vi "tsfifo_receive_canfd_msgs.vi"(7 "error in (no error)":errorcluster caption="错误输入（无错误）", 8 "Display message type":u16(ring) items=["Rx", "Rx&Tx"], 9 "AAPPChannel":u32, 10 "Path":path) -> (0 "error out":errorcluster caption="错误输出", 1 "tsfifo_receive_can_msgs":i32, 2 "ACANMsgBuffer":T1(array[cluster]), 3 "Path output":path)   [LabVIEW 2014]
doc: "Function Introduction :\nReceive FIFO CAN messages\nCall location :\ninput parameter :\nACANFDBuffers: CANFD buffers\nACANFDBuffers: canfd buffer size\nAChn: Channel Index\nARxTx: READ_TX_RX_deF_ARxTx enumeration, if the value is 0, only RX messages are received; if the value is\n1. Receive TX Rx message\nReturn value :\n0: Execution successful\nOther values: Failed"
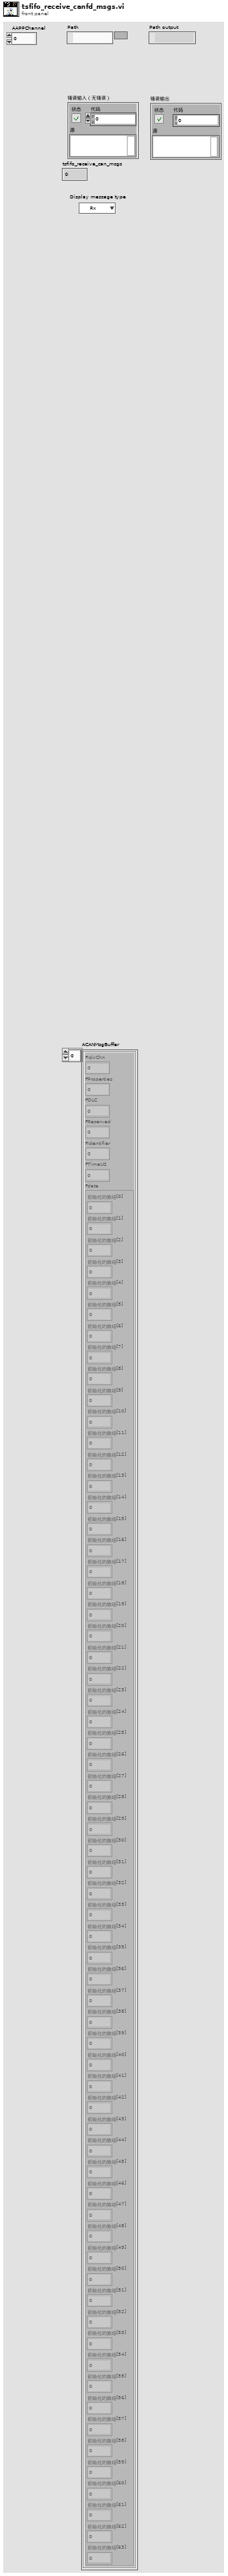
[diagram p1: front panel]
types:
  T1 = cluster{"FIdxChn":u8, "FProperties":u8, "FDLC":u8, "FReserved":u8, "FIdentifier":i32, "FTimeUS":u64, "Fdata":cluster{"初始化的数组[0]":u8, "初始化的数组[1]":u8, "初始化的数组[2]":u8, "初始化的数组[3]":u8, "初始化的数组[4]":u8, "初始化的数组[5]":u8, "初始化的数组[6]":u8, "初始化的数组[7]":u8, "初始化的数组[8]":u8, "初始化的数组[9]":u8, "初始化的数组[10]":u8, "初始化的数组[11]":u8, "初始化的数组[12]":u8, "初始化的数组[13]":u8, "初始化的数组[14]":u8, "初始化的数组[15]":u8, "初始化的数组[16]":u8, "初始化的数组[17]":u8, "初始化的数组[18]":u8, "初始化的数组[19]":u8, "初始化的数组[20]":u8, "初始化的数组[21]":u8, "初始化的数组[22]":u8, "初始化的数组[23]":u8, "初始化的数组[24]":u8, "初始化的数组[25]":u8, "初始化的数组[26]":u8, "初始化的数组[27]":u8, "初始化的数组[28]":u8, "初始化的数组[29]":u8, "初始化的数组[30]":u8, "初始化的数组[31]":u8, "初始化的数组[32]":u8, "初始化的数组[33]":u8, "初始化的数组[34]":u8, "初始化的数组[35]":u8, "初始化的数组[36]":u8, "初始化的数组[37]":u8, "初始化的数组[38]":u8, "初始化的数组[39]":u8, "初始化的数组[40]":u8, "初始化的数组[41]":u8, "初始化的数组[42]":u8, "初始化的数组[43]":u8, "初始化的数组[44]":u8, "初始化的数组[45]":u8, "初始化的数组[46]":u8, "初始化的数组[47]":u8, "初始化的数组[48]":u8, "初始化的数组[49]":u8, "初始化的数组[50]":u8, "初始化的数组[51]":u8, "初始化的数组[52]":u8, "初始化的数组[53]":u8, "初始化的数组[54]":u8, "初始化的数组[55]":u8, "初始化的数组[56]":u8, "初始化的数组[57]":u8, "初始化的数组[58]":u8, "初始化的数组[59]":u8, "初始化的数组[60]":u8, "初始化的数组[61]":u8, "初始化的数组[62]":u8, "初始化的数组[63]":u8}}[]
  T2 = cluster{"FIdxChn":u8, "FProperties":u8, "FDLC":u8, "FReserved":u8, "FIdentifier":i32, "FTimeUS":u64, "Fdata":cluster{"初始化的数组[0]":u8, "初始化的数组[1]":u8, "初始化的数组[2]":u8, "初始化的数组[3]":u8, "初始化的数组[4]":u8, "初始化的数组[5]":u8, "初始化的数组[6]":u8, "初始化的数组[7]":u8, "初始化的数组[8]":u8, "初始化的数组[9]":u8, "初始化的数组[10]":u8, "初始化的数组[11]":u8, "初始化的数组[12]":u8, "初始化的数组[13]":u8, "初始化的数组[14]":u8, "初始化的数组[15]":u8, "初始化的数组[16]":u8, "初始化的数组[17]":u8, "初始化的数组[18]":u8, "初始化的数组[19]":u8, "初始化的数组[20]":u8, "初始化的数组[21]":u8, "初始化的数组[22]":u8, "初始化的数组[23]":u8, "初始化的数组[24]":u8, "初始化的数组[25]":u8, "初始化的数组[26]":u8, "初始化的数组[27]":u8, "初始化的数组[28]":u8, "初始化的数组[29]":u8, "初始化的数组[30]":u8, "初始化的数组[31]":u8, "初始化的数组[32]":u8, "初始化的数组[33]":u8, "初始化的数组[34]":u8, "初始化的数组[35]":u8, "初始化的数组[36]":u8, "初始化的数组[37]":u8, "初始化的数组[38]":u8, "初始化的数组[39]":u8, "初始化的数组[40]":u8, "初始化的数组[41]":u8, "初始化的数组[42]":u8, "初始化的数组[43]":u8, "初始化的数组[44]":u8, "初始化的数组[45]":u8, "初始化的数组[46]":u8, "初始化的数组[47]":u8, "初始化的数组[48]":u8, "初始化的数组[49]":u8, "初始化的数组[50]":u8, "初始化的数组[51]":u8, "初始化的数组[52]":u8, "初始化的数组[53]":u8, "初始化的数组[54]":u8, "初始化的数组[55]":u8, "初始化的数组[56]":u8, "初始化的数组[57]":u8, "初始化的数组[58]":u8, "初始化的数组[59]":u8, "初始化的数组[60]":u8, "初始化的数组[61]":u8, "初始化的数组[62]":u8, "初始化的数组[63]":u8}}
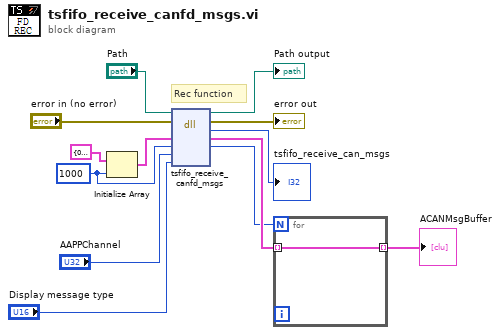
[diagram p0: block diagram]
diagram:
  w1 = 1000 ("维数大小")
  # "Rec function"
  n1 = Initialize Array(T2 {"FIdxChn"=0, "FProperties"=0, "FDLC"=0, "FReserved"=0, "FIdentifier"=0, "FTimeUS"=0, "Fdata"={"初始化的数组[0]"=0, "初始化的数组[1]"=0, "初始化的数组[2]"=0, "初始化的数组[3]"=0, "初始化的数组[4]"=0, "初始化的数组[5]"=0, "初始化的数组[6]"=0, "初始化的数组[7]"=0, "初始化的数组[8]"=0, "初始化的数组[9]"=0, "初始化的数组[10]"=0, "初始化的数组[11]"=0, "初始化的数组[12]"=0, "初始化的数组[13]"=0, "初始化的数组[14]"=0, "初始化的数组[15]"=0, "初始化的数组[16]"=0, "初始化的数组[17]"=0, "初始化的数组[18]"=0, "初始化的数组[19]"=0, "初始化的数组[20]"=0, "初始化的数组[21]"=0, "初始化的数组[22]"=0, "初始化的数组[23]"=0, "初始化的数组[24]"=0, "初始化的数组[25]"=0, "初始化的数组[26]"=0, "初始化的数组[27]"=0, "初始化的数组[28]"=0, "初始化的数组[29]"=0, "初始化的数组[30]"=0, "初始化的数组[31]"=0, "初始化的数组[32]"=0, "初始化的数组[33]"=0, "初始化的数组[34]"=0, "初始化的数组[35]"=0, "初始化的数组[36]"=0, "初始化的数组[37]"=0, "初始化的数组[38]"=0, "初始化的数组[39]"=0, "初始化的数组[40]"=0, "初始化的数组[41]"=0, "初始化的数组[42]"=0, "初始化的数组[43]"=0, "初始化的数组[44]"=0, "初始化的数组[45]"=0, "初始化的数组[46]"=0, "初始化的数组[47]"=0, "初始化的数组[48]"=0, "初始化的数组[49]"=0, "初始化的数组[50]"=0, "初始化的数组[51]"=0, "初始化的数组[52]"=0, "初始化的数组[53]"=0, "初始化的数组[54]"=0, "初始化的数组[55]"=0, "初始化的数组[56]"=0, "初始化的数组[57]"=0, "初始化的数组[58]"=0, "初始化的数组[59]"=0, "初始化的数组[60]"=0, "初始化的数组[61]"=0, "初始化的数组[62]"=0, "初始化的数组[63]"=0}} ("簇"), w1) -> (w13:T1)
  n2 = dll-call lib="PTH2@abs EDemo同星TSCAN_V1.2_20220228ConfigTSMaster.dll" fn="tsfifo_receive_canfd_msgs"(path in="Path", error in="error in (no error)", "ACANMsgBuffer"=w13, "ACANMsgBufferSize"=w1, "AChn"="AAPPChannel", "ATxRx"="Display message type") -> (path out=→"Path output":path, error out=→"error out":errorcluster, "tsfifo_receive_can_msgs"=→"tsfifo_receive_can_msgs":i32, "ACANMsgBuffer"=w4:T1, "ACANMsgBufferSize"=w3:i32)  [unwired: 3 in]
  n3 = for {
    N: w3 -> [_]
    tunnel: w4 -> [w14] mode=indexing
    tunnel: [w14] -> w2 mode=indexing
  }
  "ACANMsgBuffer" <- w2
